vi "Add.vi"(0 "object in":refnum<class "Tree.lvclass">, 2 "Value":dbl, 5 "Error In":errorcluster) -> (14 "object out":refnum<class "Tree.lvclass">, 19 "Error Out":errorcluster)   [LabVIEW 2024, in "Tree.lvclass"]
doc: "Create a new node in the tree according to given value in correct place (according to binary tree rules)"
uses:
  Tree.lvclass
  Tree.lvclass/Tree.ctl
  Node_class/Node.lvclass
panel:
  # "Connector Pane"
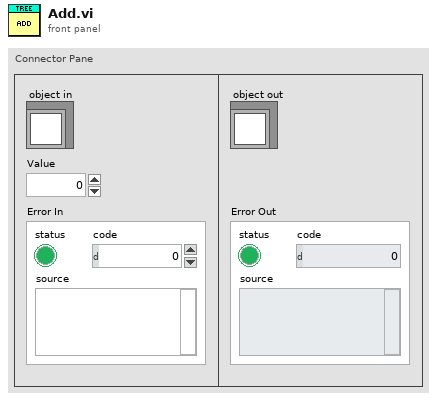
[diagram p1: front panel]
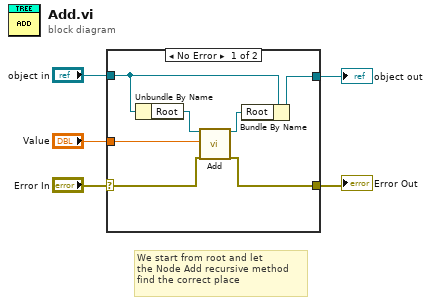
[diagram p0: block diagram]
diagram:
  # "We start from root and let\nthe Node Add recursive method\nfind the correct place"
  n1 = case shown="No Error" "Error In" {
    selector: "Error In" -> [w7 w14]
    tunnel: [w6 w14] -> w4
    tunnel: [w11 w13] -> w2
    tunnel: "object in" -> [w12 w13]
    tunnel: "Value" -> [w8 _]
    frame No Error {
      n2 = Unbundle By Name(w12) -> ("Root"=w9:refnum<class "Node.lvclass">)
      n3 = call-dynamic "Add.vi"("object in"=w9, "Value"=w8, "Error In"=w7) -> ("object out"=w10:refnum<class "Node.lvclass">, "Error Out"=w6:errorcluster)  [unwired: 15 in]
      n4 = Bundle By Name(cluster=w12, "Root"=w10) -> (w11:refnum<class "Tree.lvclass">)
    }
    frame Error {
    }
  }
  "Error Out" <- w4
  "object out" <- w2
